vi "VCI Check User Key.vi"(9 "pUserKey":dbl[](array[numeric])=[0.0, 0.0, 0.0, 0.0, 0.0, 0.0, 0.0, 0.0, 0.0, 0.0, 0.0, 0.0, 0.0, 0.0, 0.0, 0.0], 10 "DevIndex":i32, 11 "DevType":i32) -> (3 "function return":i32)   [LabVIEW 2010, in "ControlCAN.lvlib"]
doc: "int WINAPI VCI_CheckUserKey(int DevType,int DevIndex,unsigned char* pUserKey);"
uses:
  ControlCAN.lvlib
  ControlCAN/Ginkgo_Driver.dll
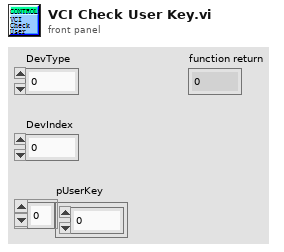
[diagram p1: front panel]
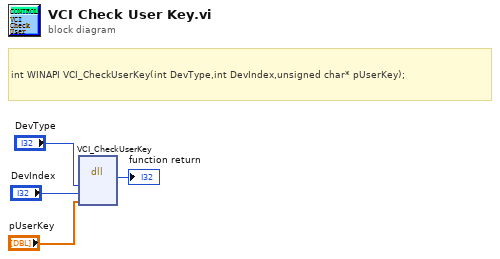
[diagram p0: block diagram]
diagram:
  # "int WINAPI VCI_CheckUserKey(int DevType,int DevIndex,unsigned char* pUserKey);"
  n1 = dll-call lib="E:/Project/vt_ginkgo/truck/Ginkgo Driver/vs2010/Ginkgo_USB-I2C&SPI&CAN_API_v2.0.3.3/lib/labview_32bit/ControlCAN/Ginkgo_Driver.*" fn="VCI_CheckUserKey"("DevType"="DevType", "DevIndex"="DevIndex", "pUserKey"="pUserKey") -> (→"function return":i32)  [unwired: 6 in, 2 out]
